vi "GCode File to Array.vi"(11 "File Path":path) -> (3 "G-Code Array":string[](array[string]))   [LabVIEW 2017]
doc: "Converts a G-Code file into a one dimensional array where each row is a G-Code command. \n\n<B>Inputs</B>: \n- File Path: G-Code file to be converted into array. \n\n<B>Outputs</B>: \n- G-Code Array: One dimensional array. Each row is a G-Code command."
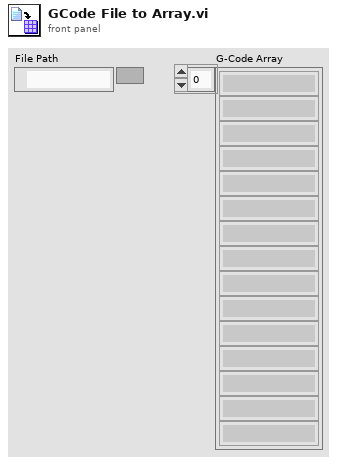
[diagram p1: front panel]
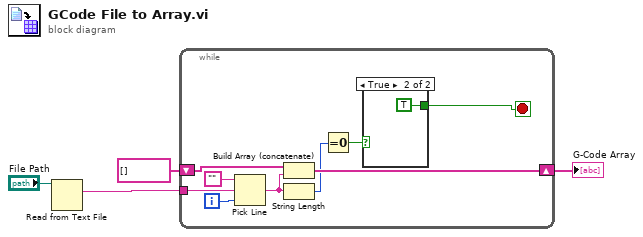
[diagram p0: block diagram]
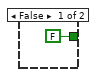
[diagram p2: hidden frame]
diagram:
  n1 = Read from Text File(file (use dialog)="File Path") -> (text=w3:string)  [unwired: 3 in, 3 out]
  n2 = while {
    shift-right: [w11] -> w2
    shift-left: string[] [] -> [w12]
    tunnel: w3 -> [w6]
    i -> [w13]
    stop <- w5 stop-if-true
    n3 = Pick Line(string ("")="", multi-line string=w6, line index=w13) -> (output string=w9:string)
    n4 = Build Array (concatenate)(w12, w9) -> (w11:string[])
    n5 = String Length(string=w9) -> (length=w8:i32)
    n6 = Equal To 0?(x=w8) -> (x = 0?=w7:bool)
    n7 = case shown="True" w7 {
      tunnel: [FALSE TRUE] -> w5
      frame False {
      }
      frame True {
      }
    }
  }
  "G-Code Array" <- w2
